vi "getClaseImagen.vi"(8 "error in":errorcluster, 11 "claseImagen in":refnum<class "claseImagen.lvclass">) -> (0 "error out":errorcluster, 2 "dataReading":T1, 3 "claseImagen out":refnum<class "claseImagen.lvclass">)   [LabVIEW 2014, in "claseImagen.lvclass"]
uses:
  claseImagen.lvclass
  claseImagen.lvclass/claseImagen.ctl
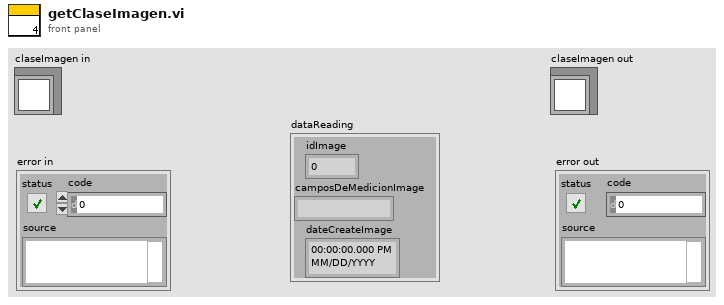
[diagram p1: front panel]
types:
  T1 = cluster{"idImage":dbl, "camposDeMedicionImage":string, "dateCreateImage":timestamp}
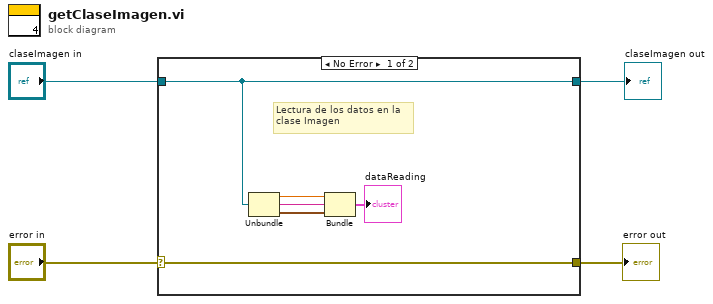
[diagram p0: block diagram]
diagram:
  n1 = case shown="No Error" "error in" {
    selector: "error in" -> [w10 w12]
    tunnel: [w10 w12] -> w3
    tunnel: "claseImagen in" -> [w5 w11]
    tunnel: [w5 w11] -> w1
    frame No Error {
      # "Lectura de los datos en la \nclase Imagen"
      n2 = Unbundle(w5) -> (w9:dbl, w8:string, w7:timestamp)
      n3 = Bundle("idImage"=w9, "camposDeMedicionImage"=w8, "dateCreateImage"=w7) -> (→"dataReading":T1)  [unwired: 1 in]
    }
    frame Error {
    }
  }
  "claseImagen out" <- w1
  "error out" <- w3
